vi "advent_1.vi"() -> ()   [LabVIEW 2021]
uses:
  <vilib>/Utility/file.llb/Read Delimited Spreadsheet (I64).vi
panel:
  out "size(s) 2":i32
  out "size(s)":i32
  out "Numeric 2":i64
  out "Numeric":i64
  out "all rows":i64[][](array[numeric])
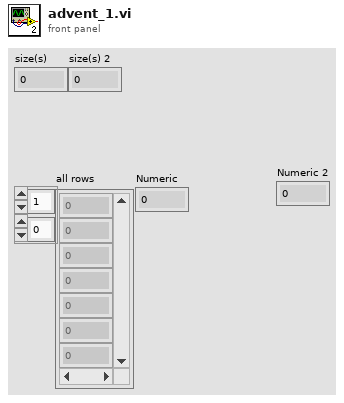
[diagram p1: front panel]
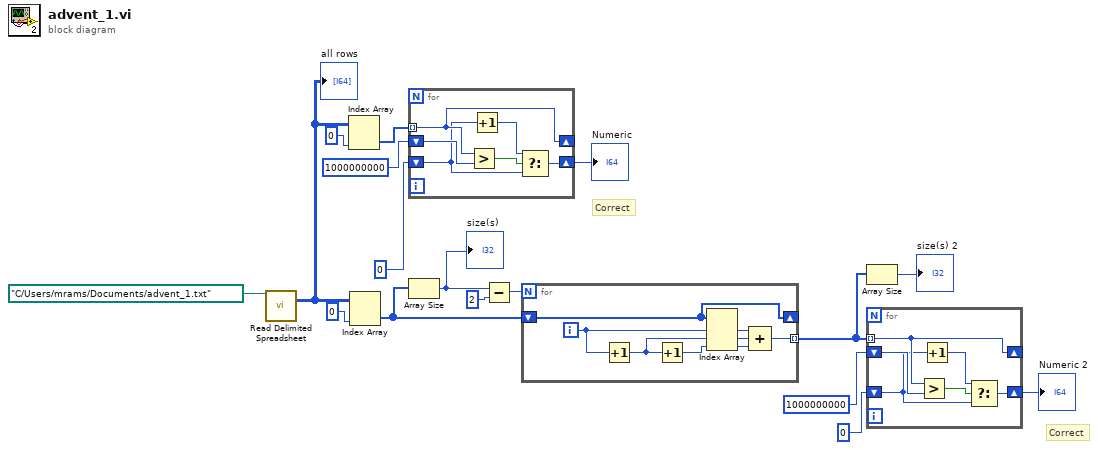
[diagram p0: block diagram]
diagram:
  # "Correct"
  # "Correct"
  n1 = call-poly <vilib>:"Read Delimited Spreadsheet.vi"("file path (dialog if empty)"=path "C:/Users/mrams/Documents/advent_1.txt") -> ("all rows"=w1:i64[][])  [unwired: 9 in, 5 out]
  "all rows" <- w1
  n2 = Index Array(array=w1, index (col)=0 ("disabled index (col)")) -> (element=w15:i64[])  [unwired: 1 in]
  n3 = Index Array(array=w1, index (col)=0 ("disabled index (col)")) -> (element=w4:i64[])  [unwired: 1 in]
  n4 = for {
    tunnel: w15 -> [w23] mode=indexing
    shift-right: [w23] -> _
    shift-left: i64 1000000000 ("Numeric") -> [w22]
    shift-right: [w18] -> w12
    shift-left: i64 0 ("Numeric") -> [w19]
    n5 = Greater?(x=w23, y=w22) -> (0:w21:bool)
    n6 = Increment(x=w19) -> (x+1=w20:i64)
    n7 = Select(t=w20, s=w21, f=w19) -> (s? t:f=w18:i64)
  }
  "Numeric" <- w12
  n8 = Array Size(array=w4) -> (size(s)=w7:i32)
  "size(s)" <- w7
  n9 = Subtract(x=w7, y=2) -> (x-y=w5:i32)
  n10 = for {
    N: w5 -> [_]
    shift-right: [w31] -> _
    shift-left: w4 -> [w31]
    tunnel: [w24] -> w2 mode=indexing
    i -> [w30]
    n11 = Increment(x=w30) -> (x+1=w29:i32)
    n12 = Increment(x=w29) -> (x+1=w28:i32)
    n13 = Index Array(array=w31, index #1=w30, index #2=w29, index #3=w28) -> (element #1=w27:i64, element #2=w26:i64, element #3=w25:i64)
    n14 = Compound Arithmetic op=ADD(w27, w26, w25) -> (w24:i64)
  }
  n15 = Array Size(array=w2) -> (size(s)=→"size(s) 2":i32)
  n16 = for {
    tunnel: w2 -> [w37] mode=indexing
    shift-right: [w37] -> _
    shift-left: i64 1000000000 ("Numeric") -> [w36]
    shift-right: [w32] -> w11
    shift-left: i64 0 ("Numeric") -> [w33]
    n17 = Greater?(x=w37, y=w36) -> (0:w35:bool)
    n18 = Increment(x=w33) -> (x+1=w34:i64)
    n19 = Select(t=w34, s=w35, f=w33) -> (s? t:f=w32:i64)
  }
  "Numeric 2" <- w11
